vi "fl28x Revision Query.vi"(8 "error in (no error)":errorcluster, 11 "VISA session":refnum<visa-resource-name>) -> (0 "error out":errorcluster, 1 "Instr Firmware Revision":string, 2 "Instrument Name":string, 3 "dup VISA session":refnum<visa-resource-name>, 4 "Modelo":string, 5 "Fabricante":string)   [LabVIEW 2015, in "289.lvclass"]
doc: "This VI queries the current instrument firmware revision and instrument driver revision.\n\nThis Instrument Driver's Revision number is \"REV 1.0, 01/2003, LV 6.1\" and is compatible with Instrument Firmware Revision V2.02\n\nFLUKE 187, 189 Digital Multimeters\nCreated By: Tom Brass, Seagate Technology \nPH. 952-402-2118\nEmail: Tom.J.Brass@Seagate.Com"
uses:
  289.lvclass
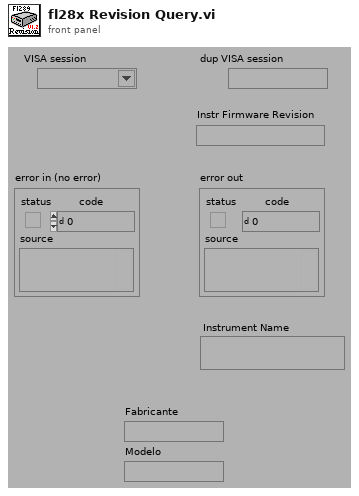
[diagram p1: front panel]
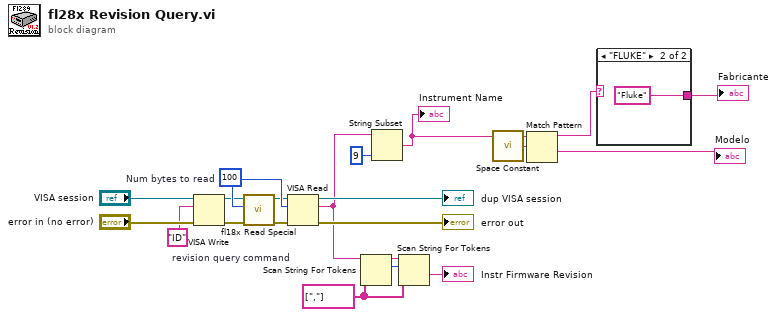
[diagram p0: block diagram]
diagram:
  w13 = string[] [","] ("delimiters (\\s,\\t,\\r,\\n)")
  w17 = "ID"  # revision query command
  w16 = u32 100  # Num bytes to read
  n1 = VISA Write(VISA resource name="VISA session", write buffer=w17, error in (no error)="error in (no error)") -> (VISA resource name out=w11:refnum<visa-resource-name>, error out=w8:errorcluster)  [unwired: 1 out]
  n2 = call <instrlib>:"fl18x Read Special.vi"("error in (no error)"=w8, "Byte Count (0)"=w16, "VISA session"=w11) -> ("error out"=w9:errorcluster, "dup VISA session"=w10:refnum<visa-resource-name>)  [unwired: 6 in, 1 out]
  n3 = VISA Read(VISA resource name=w10, byte count=w16, error in (no error)=w9) -> (VISA resource name out=→"dup VISA session":refnum<visa-resource-name>, read buffer=w7:string, error out=→"error out":errorcluster)  [unwired: 1 out]
  n4 = Scan String For Tokens(6:w13, 9:w7) -> (2:w14:i32, 3:w15:string)  [unwired: 4 in, 2 out]
  n5 = String Subset(string=w7, length (rest)=9 ("length (rest)")) -> (substring=w5:string)  [unwired: 1 in]
  "Instrument Name" <- w5
  n6 = Scan String For Tokens(6:w13, 8:w14, 9:w15) -> (1:→"Instr Firmware Revision":string)  [unwired: 3 in, 3 out]
  n7 = call <vilib>:"Space Constant.vi"() -> ("String"=w4:string)
  n8 = Match Pattern(string=w5, regular expression=w4) -> (before substring=w3:string, after substring=→"Modelo":string)  [unwired: 1 in, 2 out]
  n9 = case shown="\"FLUKE\"" w3 {
    tunnel: [_ "Fluke" ("Fabricante")] -> w2
    frame "False", Default {
    }
    frame "FLUKE" {
    }
  }
  "Fabricante" <- w2
